vi "外观 1.vi"(0 "Data In":T5 caption="数据输入", 2 "Display State In":T3 caption="显示状态输入", 3 "Container State":T4 caption="容器状态") -> (6 "Data Out":T5 caption="数据输出", 7 "Display State Out":T3 caption="显示状态输出", 8 "Action":T2 caption="动作")   [LabVIEW 2016, in "质控单元.lvlib" / "质控24H周期设置.xctl"]
uses:
  <vilib>/_xctls/Container State.ctl
  <vilib>/_xctls/Action.ctl
  <vilib>/_xctls/XControlSupport.lvlib
panel:
  in  "簇":T1
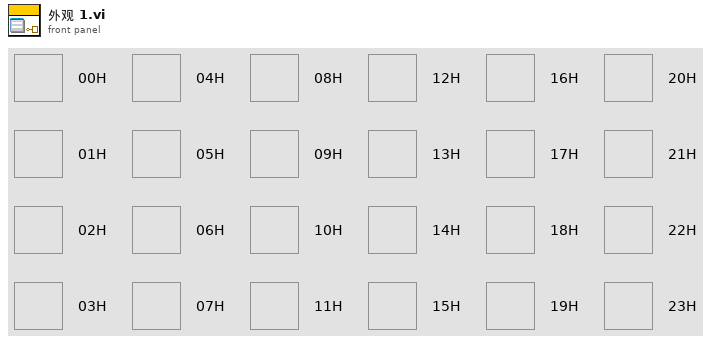
[diagram p1: front panel]
types:
  T1 = cluster{"00H":bool, "01H":bool, "02H":bool, "03H":bool, "04H":bool, "05H":bool, "06H":bool, "07H":bool, "08H":bool, "09H":bool, "10H":bool, "11H":bool, "12H":bool, "13H":bool, "14H":bool, "15H":bool, "16H":bool, "17H":bool, "18H":bool, "19H":bool, "20H":bool, "21H":bool, "22H":bool, "23H":bool}
  T2 = typedef "XControlSupport.lvlib/Action.ctl" = cluster{"Data Changed?":bool, "State Changed?":bool, "Action Name":string}
  T3 = typedef "质控单元.lvlib/质控24H周期设置.xctl/状态 1.ctl" = cluster{"Numeric":dbl}
  T4 = typedef "XControlSupport.lvlib/Container State.ctl" = cluster{"Indicator?":bool, "Run Mode?":bool, " Refnum":refnum<vi>}
  T5 = typedef "质控单元.lvlib/质控24H周期设置.xctl/数据 1.ctl" = bool[]
  T6 = cluster{"Data In[0]":bool, "Data In[1]":bool, "Data In[2]":bool, "Data In[3]":bool, "Data In[4]":bool, "Data In[5]":bool, "Data In[6]":bool, "Data In[7]":bool, "Data In[8]":bool, "Data In[9]":bool, "Data In[10]":bool, "Data In[11]":bool, "Data In[12]":bool, "Data In[13]":bool, "Data In[14]":bool, "Data In[15]":bool, "Data In[16]":bool, "Data In[17]":bool, "Data In[18]":bool, "Data In[19]":bool, "Data In[20]":bool, "Data In[21]":bool, "Data In[22]":bool, "Data In[23]":bool}
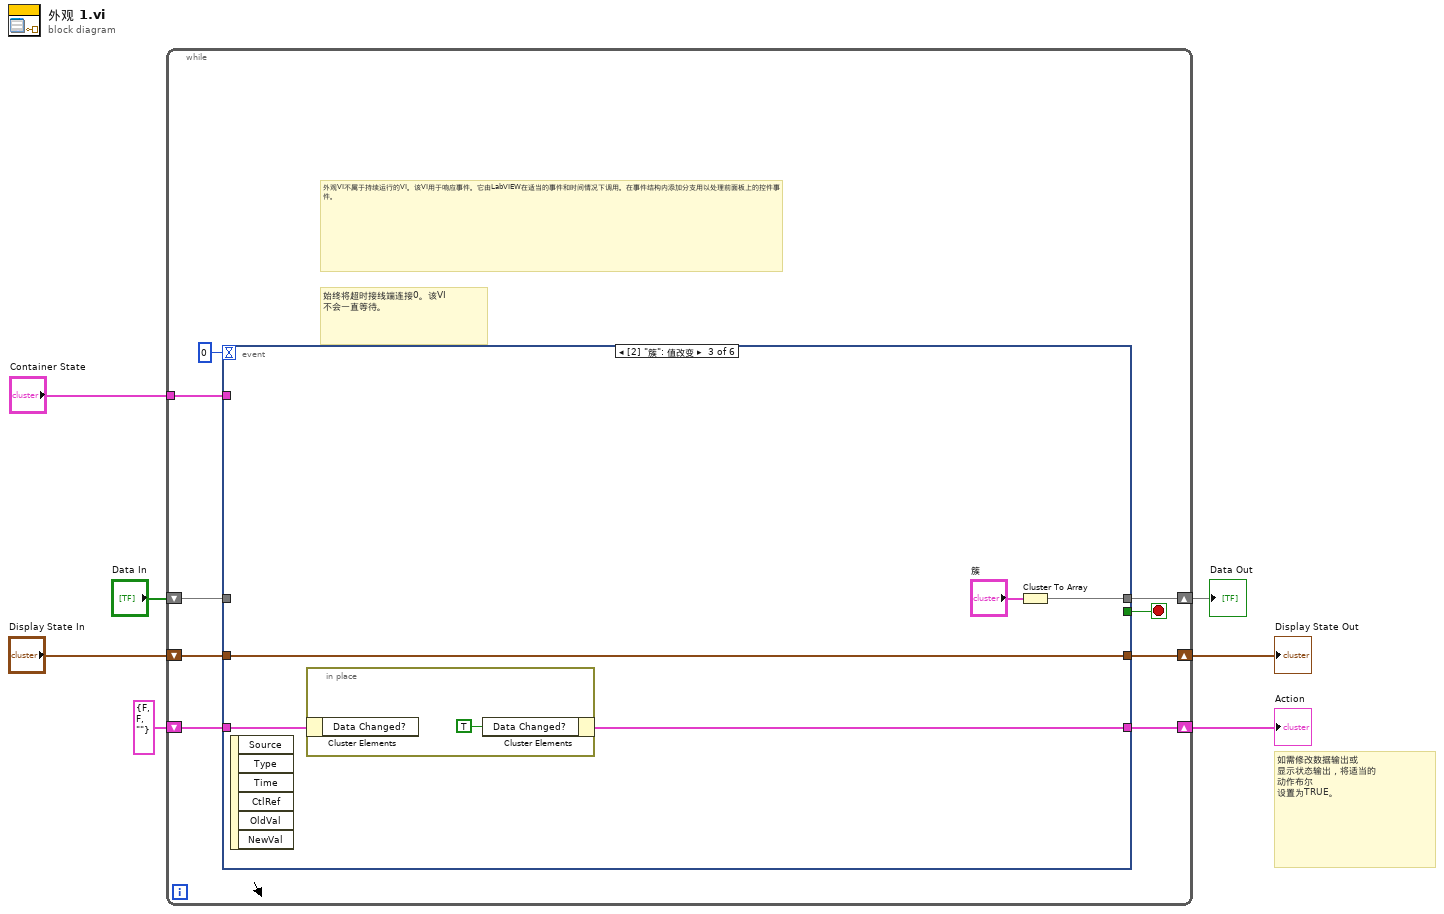
[diagram p0: block diagram]
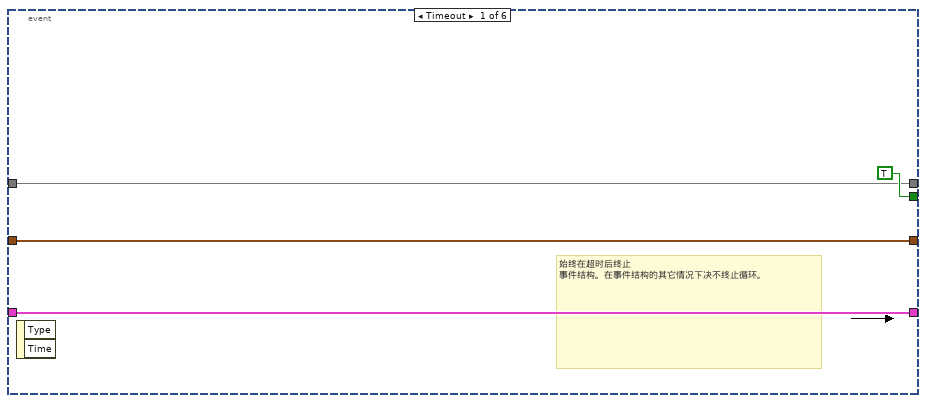
[diagram p2: hidden frame]
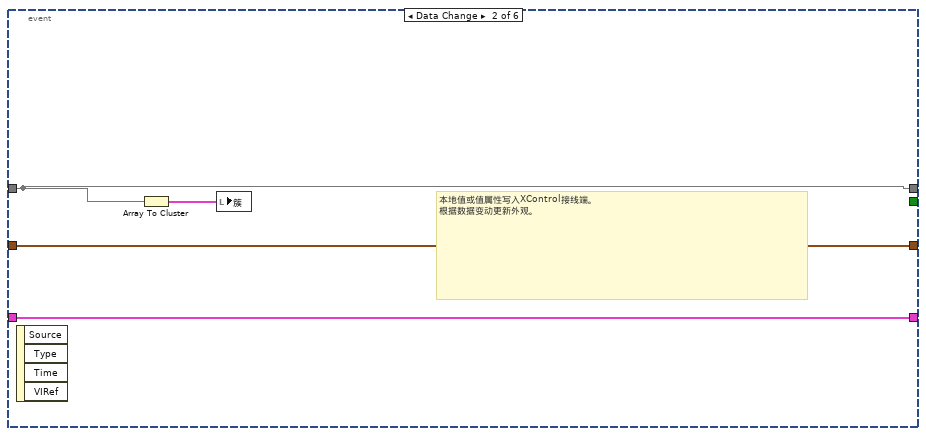
[diagram p3: hidden frame]
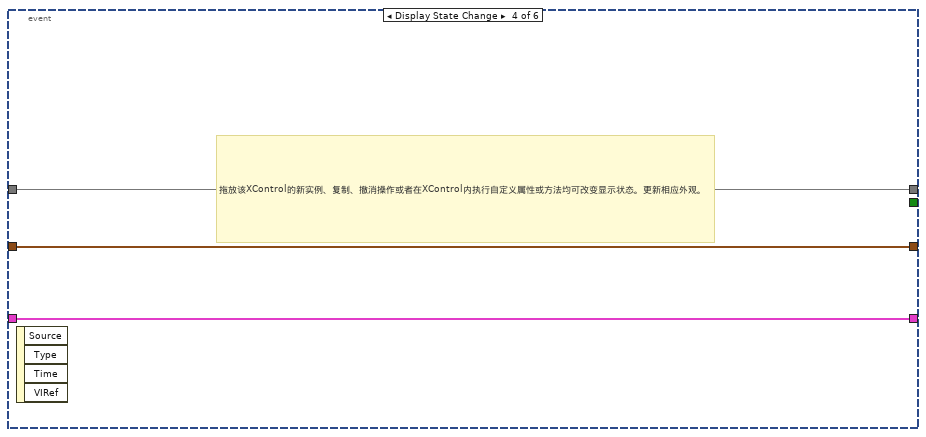
[diagram p4: hidden frame]
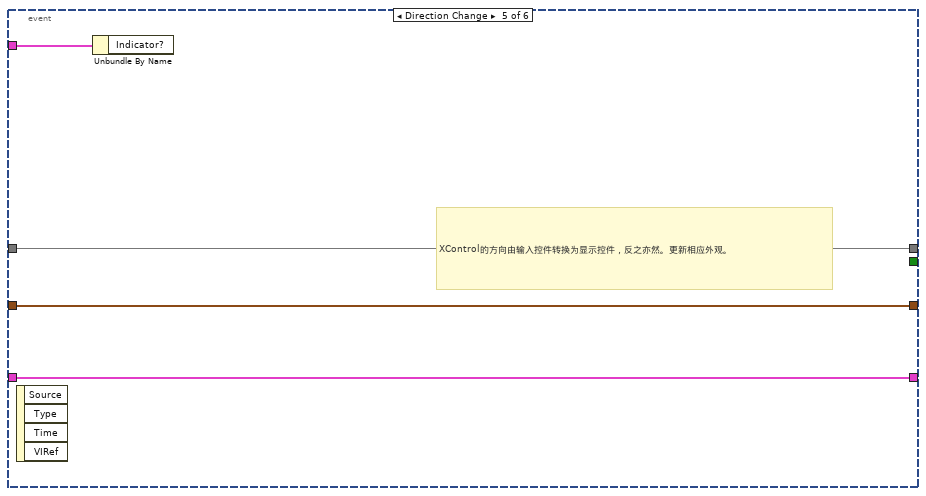
[diagram p5: hidden frame]
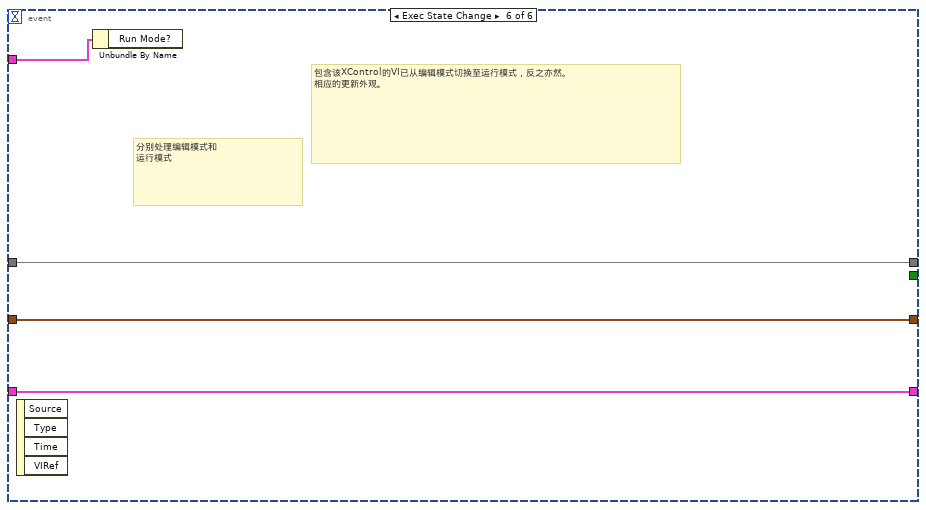
[diagram p6: hidden frame]
diagram:
  # "如需修改数据输出或\n显示状态输出，将适当的\n动作布尔\n设置为TRUE。"
  n1 = while {
    shift-right: [w15] -> w4
    shift-left: "Display State In" -> [w16]
    tunnel: "Container State" -> [w12]
    shift-right: [w10] -> w7
    shift-left: "Data In" -> [w11]
    shift-right: [w8] -> w2
    shift-left: T2 {"Data Changed?"=FALSE, "State Changed?"=FALSE, "Action Name"=""} ("Action") -> [w9]
    stop <- w14 stop-if-true
    # "外观VI不属于持续运行的VI。该VI用于响应事件。它由LabVIEW在适当的事件和时间情况下调用。在事件结构内添加分支用以处理前面板上的控件事件。"
    # "始终将超时接线端连接0。该VI\n不会一直等待。"
    n2 = event shown="[2] \"簇\": 值改变" {
      selector: _ -> [_ _ _ _ _ _]
      dyn-events: _ -> [_ _ _ _ _ _]
      timeout: 0 -> [_ _ _ _ _ _]
      tunnel: w16 -> [w18 w24 w29 w33 w36 w40]
      tunnel: [w18 w24 w29 w33 w36 w40] -> w15
      tunnel: [TRUE _ _ _ _ _] -> w14
      tunnel: w12 -> [_ _ _ _ w37 w41]
      tunnel: w11 -> [w17 w22 _ w32 w35 w39]
      tunnel: [w17 w22 w25 w32 w35 w39] -> w10
      tunnel: [w19 w23 w27 w31 w34 w38] -> w8
      tunnel: w9 -> [w19 w23 w28 w31 w34 w38]
      event Timeout {
        # "始终在超时后终止\n事件结构。在事件结构的其它情况下决不终止循环。"
        n3 = event-data() -> ()  [unwired: 1 in, 2 out]
      }
      event Data Change {
        # "本地值或值属性写入XControl接线端。\n根据数据变动更新外观。"
        n4 = event-data() -> ()  [unwired: 1 in, 4 out]
        n5 = Array To Cluster(array=w22) -> (cluster=w21:T6)
        n6 = local write "簇"(w21) -> ()
      }
      event "簇": Value Change {
        n7 = event-data() -> ()  [unwired: 1 in, 6 out]
        n8 = in-place {
          n9 = in-place-cluster #1(w28) -> ()  [unwired: 1 out]
          n10 = in-place-cluster #1("Data Changed?"=TRUE) -> (w27:T2)
        }
        n11 = Cluster To Array(cluster="簇") -> (array=w25:bool[])
      }
      event Display State Change {
        # "拖放该XControl的新实例、复制、撤消操作或者在XControl内执行自定义属性或方法均可改变显示状态。更新相应外观。"
        n12 = event-data() -> ()  [unwired: 1 in, 4 out]
      }
      event Direction Change {
        # "XControl的方向由输入控件转换为显示控件，反之亦然。更新相应外观。"
        n13 = event-data() -> ()  [unwired: 1 in, 4 out]
        n14 = Unbundle By Name(w37) -> ()  [unwired: 1 out]
      }
      event Exec State Change {
        # "包含该XControl的VI已从编辑模式切换至运行模式，反之亦然。\n相应的更新外观。"
        # "分别处理编辑模式和\n运行模式"
        n15 = event-data() -> ()  [unwired: 1 in, 4 out]
        n16 = Unbundle By Name(w41) -> ()  [unwired: 1 out]
      }
    }
  }
  "Display State Out" <- w4
  "Data Out" <- w7
  "Action" <- w2
